vi "游标显示-归零试验.vi"(3 "计算参数 in":T2, 5 "reference in":refnum<vi>) -> (0 "计算参数 out":T2, 2 "reference out":refnum<vi>)   [LabVIEW 2013]
panel:
  in  "Array":string[](array[string])=["行程", "油压1"]
  out "Yrange":dbl
  out "Xrange":dbl
  in  "Cursor":T1
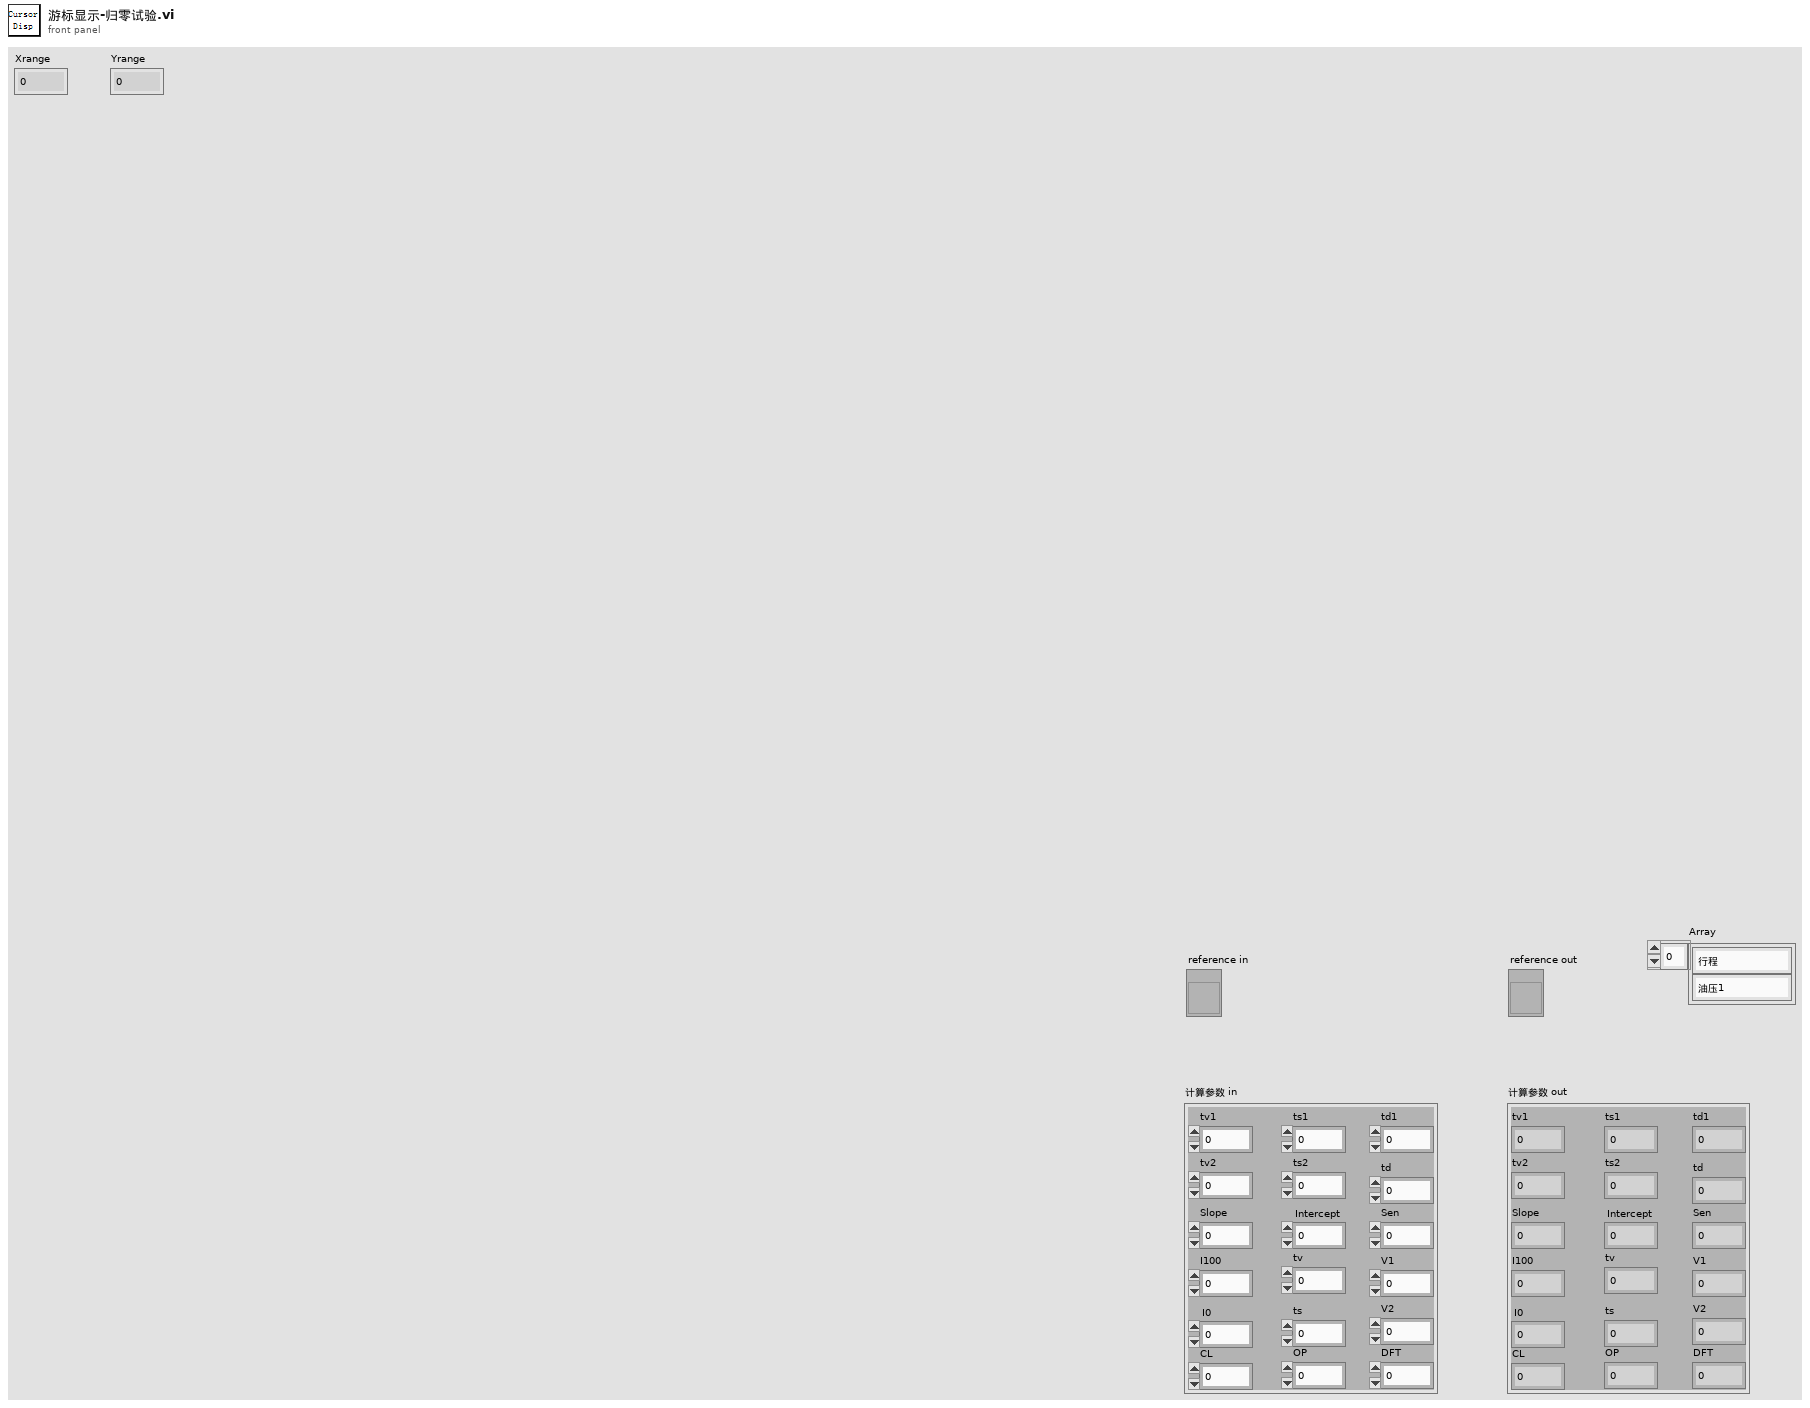
[diagram p1: front panel]
types:
  T1 = cluster{"Name":string, "Color":u32, "Style":u8, "Point Style":u8, "Name Visible":bool, "Allow Drag":bool, "Cursor Mode":u32, "Plot":i32, "Index":i32, "Position":cluster{"X":dbl, "Y":dbl}, "X Scale":u32, "Y Scale":u32, "Watch Plots":i32[], "Watch All Plots":bool, "Plot Area":i32, "Label Offset":cluster{"X":dbl, "Y":dbl}}
  T2 = cluster{"tv1":dbl, "tv2":dbl, "tv":dbl, "ts1":dbl, "ts2":dbl, "ts":dbl, "td1":dbl, "td":dbl, "Slope":dbl, "Intercept":dbl, "I100":dbl, "I0":dbl, "Sen":dbl, "V1":dbl, "V2":dbl, "CL":dbl, "OP":dbl, "DFT":dbl}
  T3 = cluster{"Name":string, "Color":u32, "Style":u8, "Point Style":u8, "Name Visible":bool, "Allow Drag":bool, "Cursor Mode":u32, "Plot":i32, "Index":i32, "Position":cluster{"X":dbl, "Y":dbl}, "X Scale":u32, "Y Scale":u32, "Watch Plots":i32[], "Watch All Plots":bool, "Plot Area":i32, "Label Offset":cluster{"X":dbl, "Y":dbl}}[]
  T4 = typedef "LVCursorListTypeDef.ctl" = cluster{"Name":string, "Color":u32, "Style":u8, "Point Style":u8, "Name Visible":bool, "Allow Drag":bool, "Cursor Mode":u32, "Plot":i32, "Index":i32, "Position":cluster{"X":dbl, "Y":dbl}, "X Scale":u32, "Y Scale":u32, "Watch Plots":i32[], "Watch All Plots":bool, "Plot Area":i32, "Label Offset":cluster{"X":dbl, "Y":dbl}}[]
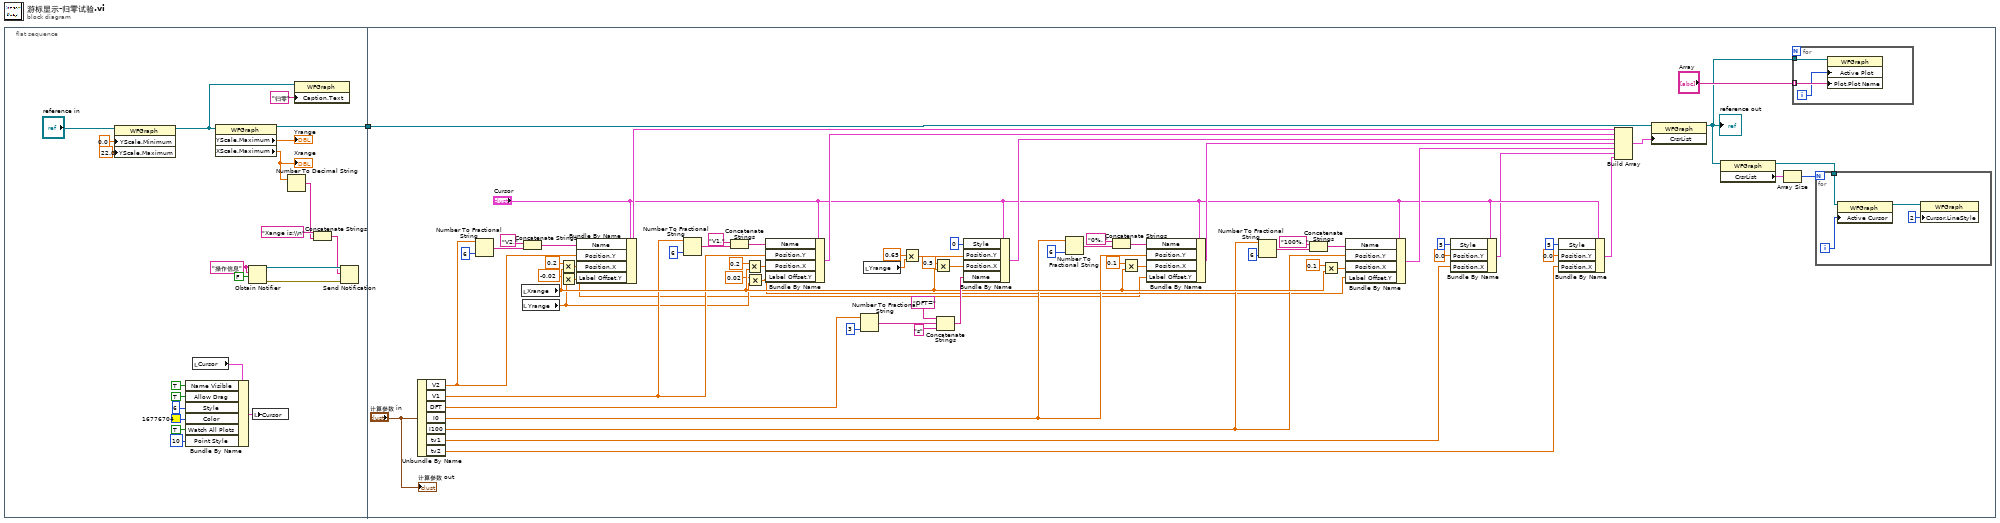
[diagram p0: block diagram]
diagram:
  n1 = flat-sequence {
    tunnel: [w16] -> w1
    tunnel: w1 -> [w46]
    frame #0 {
      w9 = "操作信息" ("name (unnamed)")
      n2 = property class="WFGraph"(reference="reference in", "YScale.Minimum"=0.0 ("Y Scale.Range:Minimum"), "YScale.Maximum"=22.0 ("Y Scale.Range:Maximum")) -> (reference out=w12:refnum<vi>)  [unwired: 1 in, 1 out]
      n3 = local read "Cursor"() -> (w21:T1)
      n4 = Bundle By Name(cluster=w21, "Name Visible"=TRUE, "Allow Drag"=TRUE, "Style"=u8 6, "Color"=u32 16776704, "Watch All Plots"=TRUE, "Point Style"=u8 10) -> (w20:T1)
      n5 = property class="WFGraph"(reference=w12) -> (reference out=w16:refnum<vi>, "YScale.Maximum"=→"Yrange":dbl, "XScale.Maximum"=w4:dbl)  [unwired: 1 in, 1 out]
      "Xrange" <- w4
      n6 = Obtain Notifier(name (unnamed)=w9, notification data type=w9, create if not found? (T)=FALSE) -> (notifier out=w7:refnum<notifier>, error out=w6:errorcluster)  [unwired: 1 in, 1 out]
      n7 = local write "Cursor"(w20) -> ()
      n8 = Number To Decimal String(number=w4) -> (decimal integer string=w3:string)  [unwired: 1 in]
      n9 = property on="Property Node" class="WFGraph"(reference=w12, "Caption.Text"="归零") -> ()  [unwired: 1 in, 2 out]
      n10 = Concatenate Strings("Xange is:\\n", w3) -> (w2:string)
      n11 = Send Notification(notification=w2, notifier=w7, error in (no error)=w6) -> ()  [unwired: 2 out]
    }
    frame #1 {
      n12 = Unbundle By Name("计算参数 in") -> ("V2"=w47:dbl, "V1"=w48:dbl, "DFT"=w92:dbl, "I0"=w36:dbl, "I100"=w35:dbl, "tv1"=w40:dbl, "tv2"=w39:dbl)
      n13 = Number To Fractional String(number=w47, precision (6)=i16 6 ("宽度(-)")) -> (F-format string=w73:string)  [unwired: 2 in]
      n14 = local read "Xrange"() -> (w49:dbl)
      n15 = local read "Yrange"() -> (w28:dbl)
      n16 = Concatenate Strings("V2," ("光标.游标名"), w73) -> (w65:string)
      n17 = Multiply(x=0.2 ("y"), y=w49) -> (x*y=w64:dbl)
      n18 = Multiply(x=-0.02 ("y"), y=w28) -> (x*y=w27:dbl)
      n19 = Bundle By Name(cluster="Cursor", "Name"=w65, "Position.Y"=w47, "Position.X"=w64, "Label Offset.Y"=w27) -> (w91:T1)
      n20 = Number To Fractional String(number=w48, precision (6)=i16 6 ("宽度(-)")) -> (F-format string=w76:string)  [unwired: 2 in]
      n21 = Concatenate Strings("V1," ("光标.游标名"), w76) -> (w78:string)
      n22 = Multiply(x=0.2 ("y"), y=w49) -> (x*y=w79:dbl)
      n23 = Multiply(x=0.02 ("y"), y=w28) -> (x*y=w30:dbl)
      n24 = Bundle By Name(cluster="Cursor", "Name"=w78, "Position.Y"=w48, "Position.X"=w79, "Label Offset.Y"=w30) -> (w90:T1)
      n25 = Number To Fractional String(number=w92, precision (6)=i16 3 ("宽度(-)")) -> (F-format string=w52:string)  [unwired: 2 in]
      n26 = local read "Yrange"() -> (w59:dbl)
      n27 = Multiply(x=0.65 ("y"), y=w59) -> (x*y=w61:dbl)
      n28 = Multiply(x=0.5 ("y"), y=w49) -> (x*y=w83:dbl)
      n29 = Concatenate Strings("DFT=" ("字符串"), w52, "s" ("字符串")) -> (w85:string)
      n30 = Bundle By Name(cluster="Cursor", "Style"=u8 0, "Position.Y"=w61, "Position.X"=w83, "Name"=w85) -> (w89:T1)
      n31 = Number To Fractional String(number=w36, precision (6)=i16 6 ("宽度(-)")) -> (F-format string=w70:string)  [unwired: 2 in]
      n32 = Concatenate Strings("0%, " ("光标.游标名"), w70) -> (w62:string)
      n33 = Multiply(x=0.1 ("y"), y=w49) -> (x*y=w57:dbl)
      n34 = Bundle By Name(cluster="Cursor", "Name"=w62, "Position.Y"=w36, "Position.X"=w57, "Label Offset.Y"=w27) -> (w88:T1)
      n35 = Number To Fractional String(number=w35, precision (6)=i16 6 ("宽度(-)")) -> (F-format string=w67:string)  [unwired: 2 in]
      n36 = Concatenate Strings("100%, " ("光标.游标名"), w67) -> (w63:string)
      n37 = Multiply(x=0.1 ("y"), y=w49) -> (x*y=w55:dbl)
      n38 = Bundle By Name(cluster="Cursor", "Name"=w63, "Position.Y"=w35, "Position.X"=w55, "Label Offset.Y"=w30) -> (w87:T1)
      n39 = Bundle By Name(cluster="Cursor", "Style"=u8 5, "Position.Y"=0.0, "Position.X"=w40) -> (w41:T1)
      n40 = Bundle By Name(cluster="Cursor", "Style"=u8 5, "Position.Y"=0.0, "Position.X"=w39) -> (w42:T1)
      n41 = Build Array(w91, w90, w89, w88, w87, w41, w42) -> (w86:T3)
      n42 = property class="WFGraph"(reference=w46, "CrsrList"=w86) -> (reference out=w25:refnum<vi>)  [unwired: 1 in, 1 out]
      "reference out" <- w25
      n43 = property class="WFGraph"(reference=w25) -> (reference out=w32:refnum<vi>, "CrsrList"=w34:T4)  [unwired: 1 in, 1 out]
      n44 = Array Size(array=w34) -> (size(s)=w33:i32)
      n45 = for {
        tunnel: "Array" -> [w95] mode=indexing
        tunnel: w25 -> [w94]
        i -> [w93]
        n46 = property class="WFGraph"(reference=w94, "Active Plot"=w93, "Plot.Plot Name"=w95) -> ()  [unwired: 1 in, 2 out]
      }
      n47 = for {
        N: w33 -> [_]
        tunnel: w32 -> [w99]
        i -> [w98]
        n48 = property class="WFGraph"(reference=w99, "Active Cursor"=w98) -> (reference out=w97:refnum<vi>)  [unwired: 1 in, 1 out]
        n49 = property class="WFGraph"(reference=w97, "Cursor.LineStyle"=u8 2 ("Cursor.Line Style")) -> ()  [unwired: 1 in, 2 out]
      }
      "计算参数 out" <- "计算参数 in"
    }
  }
